vi "HMAC-SHA256.vi"(7 "Key":string, 8 "error In":errorcluster, 11 "String to Encode":string) -> (0 "error Out":errorcluster, 3 "Hash String":string)   [LabVIEW 2012, in "SHA256.lvlib"]
doc: "Calculates the SHA256 HMAC signature"
uses:
  SHA256.lvlib
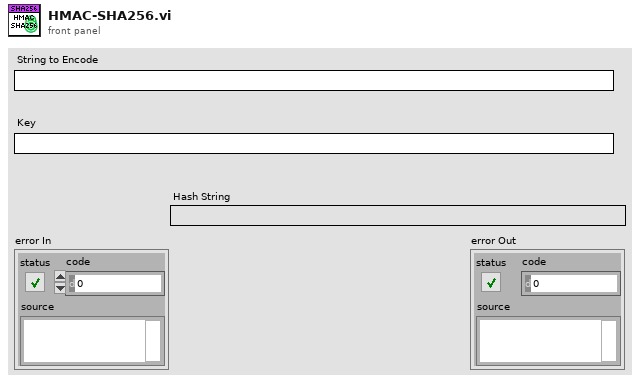
[diagram p1: front panel]
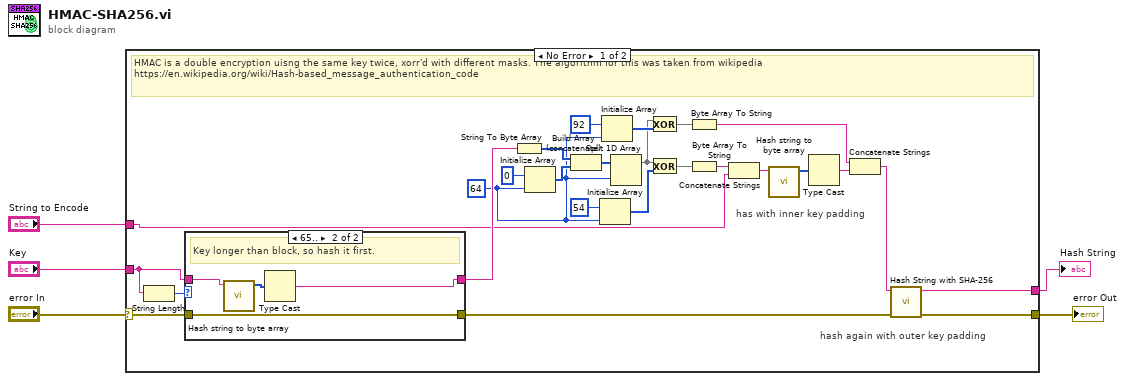
[diagram p0: block diagram]
diagram:
  n1 = case shown="No Error" "error In" {
    selector: "error In" -> [w29 w38]
    tunnel: "Key" -> [w30 _]
    tunnel: "String to Encode" -> [w16 _]
    tunnel: [w13 w38] -> w2
    tunnel: [w12 _] -> w1
    frame No Error {
      w9 = 64 ("dimension size")
      # "hash again with outer key padding"
      # "has with inner key padding"
      # "HMAC is a double encryption uisng the same key twice, xorr'd with different masks. The algorithm for this was taken from wikipedia \nhttps://en.wikipedia.org/wiki/Hash-based_message_authentication_code"
      n2 = String Length(string=w30) -> (length=w31:i32)
      n3 = case shown="65.." w31 {
        tunnel: w30 -> [w33 w37]
        tunnel: w29 -> [w32 w36]
        tunnel: [w32 w36] -> w11
        tunnel: [w33 w35] -> w28
        frame 0, Default {
        }
        frame 65.. {
          # "Key longer than block, so hash it first."
          n4 = call "Hash string to byte array.vi"("String to Encode"=w37) -> ("H Array"=w34:u32[])  [unwired: 10 in]
          n5 = Type Cast(x=w34) -> (*(type *) &x=w35:string)  [unwired: 1 in]
        }
      }
      n6 = String To Byte Array(string=w28) -> (unsigned byte array=w27:u8[])
      n7 = Initialize Array(u8 0 ("element"), w9) -> (w25:u8[])
      n8 = Build Array (concatenate)(w27, w25) -> (w24:u8[])
      n9 = Initialize Array(u8 54, w9) -> (w20:u8[])
      n10 = Initialize Array(u8 92, w9) -> (w21:u8[])
      n11 = Split 1D Array(array=w24, index=w9) -> (first subarray=w19:u8[])  [unwired: 1 out]
      n12 = Exclusive Or(1:w21, 2:w19) -> (0:w18:u8[])
      n13 = Exclusive Or(1:w20, 2:w19) -> (0:w17:u8[])
      n14 = Byte Array To String(unsigned byte array=w18) -> (string=w15:string)
      n15 = Byte Array To String(unsigned byte array=w17) -> (string=w10:string)
      n16 = Concatenate Strings(w10, w16) -> (w8:string)
      n17 = call "Hash string to byte array.vi"("String to Encode"=w8) -> ("H Array"=w7:u32[])  [unwired: 10 in]
      n18 = Type Cast(x=w7) -> (*(type *) &x=w6:string)  [unwired: 1 in]
      n19 = Concatenate Strings(w15, w6) -> (w14:string)
      n20 = call "Hash String with SHA-256.vi"("error In"=w11, "String to Encode"=w14) -> ("error Out"=w13:errorcluster, "Hash String"=w12:string)  [unwired: 8 in]
    }
    frame Error {
    }
  }
  "Hash String" <- w1
  "error Out" <- w2
